vi "Vision Processing.vi"(4 "error in (no error)":errorcluster) -> ()   [LabVIEW 2012]
doc: "This VI runs in parallel to other tasks. It gets images from the camera, processes them for color or shape and use that information to affect robot behavior."
uses:
  Robot Global Data.vi
  Vision Global Data.vi
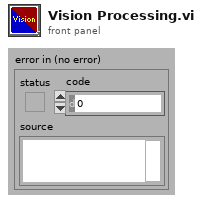
[diagram p1: front panel]
types:
  T1 = typedef "Image Type" = u32
  T2 = typedef "WPI_CameraDevRef.ctl" = cluster{"Camera Address":string, "CameraStatus":errorcluster, "Acquire Image Notifier":refnum<notifier>}
  T3 = typedef "IMAQ Image.ctl" = refnum<image>
  T4 = typedef "TargetData.ctl" = cluster{"X":dbl, "Y":dbl, "Z":dbl}
  T5 = typedef "WPI_CameraImageSize.ctl" = enum16{"640x480", "320x240", "160x120"}
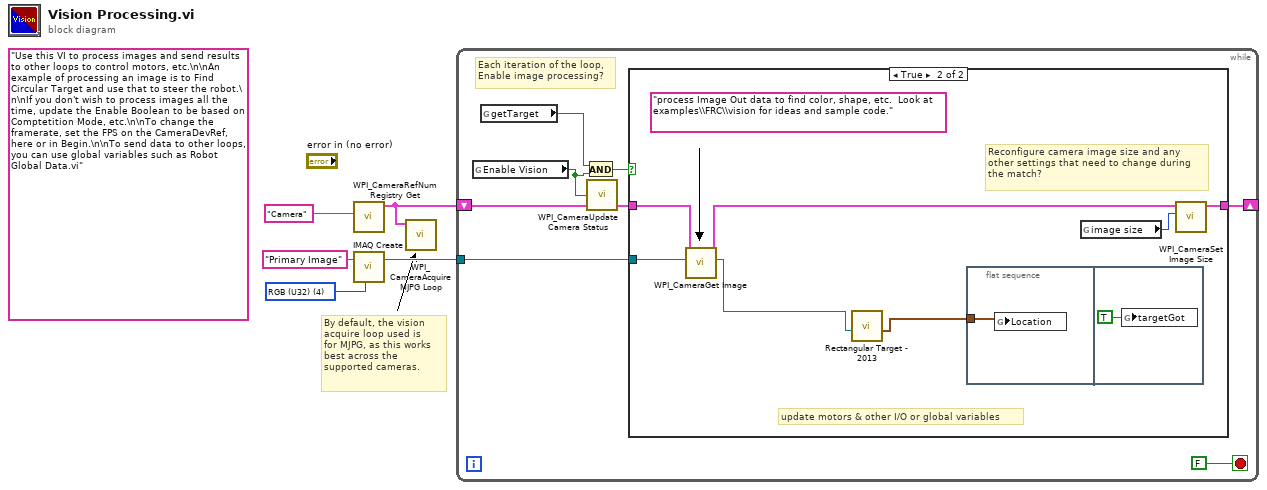
[diagram p0: block diagram]
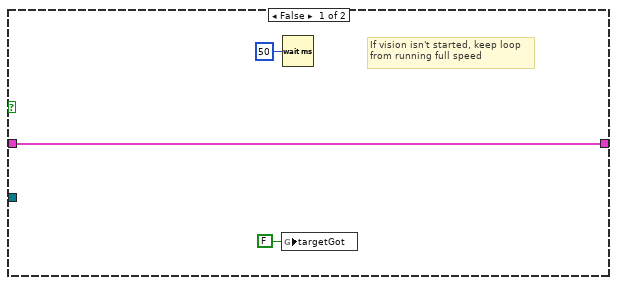
[diagram p2: hidden frame]
diagram:
  (unwired) "Use this VI to process images and send results to other loops to control motors, etc.\n\nAn example of processing an image is to Find Circular Target and use that to steer the robot.\n\nIf you don't wish to process images all the time, update the Enable Boolean to be based on Comptetition Mode, etc.\n\nTo change the framerate, set the FPS on the CameraDevRef, here or in Begin.\n\nTo send data to other loops, you can use global variables such as Robot Global Data.vi"
  w5 = T1 4 items=["Grayscale (U8)", "Grayscale (I16)", "Grayscale (SGL)", "Complex (CSG)", "RGB (U32)", "HSL (U32)", "RGB (U64)"] ("Image Type")
  # "By default, the vision\nacquire loop used is\nfor MJPG, as this works\nbest across the\nsupported cameras."
  n1 = call <vilib>:"WPI_CameraRefNum Registry Get.vi"("refnum name"="Camera") -> ("CameraDevRef"=w1:T2)  [unwired: 1 in, 9 out]
  n2 = call "IMAQ Create"("Image Name"="Primary Image", "Image Type"=w5) -> ("New Image"=w3:T3)  [unwired: 2 in, 2 out]
  n3 = call <vilib>:"WPI_CameraAcquire MJPG Loop.vi"("CameraDevRef"=w1) -> ()  [unwired: 11 in]
  n4 = while {
    shift-right: [w12] -> _
    shift-left: w1 -> [w10]
    tunnel: w3 -> [w11]
    stop <- FALSE stop-if-true
    # "Each iteration of the loop,\nEnable image processing?"
    n5 = global read "Robot Global Data.vi" "Enable Vision"() -> (w6:bool)
    n6 = global read "Vision Global Data.vi" "getTarget"() -> (w7:bool)
    n7 = And(x=w7, y=w6) -> (x .and. y?=w8:bool)
    n8 = call <vilib>:"WPI_CameraUpdate Camera Status.vi"("CameraDevRef In"=w10, "Enable Vision"=w6) -> ("CameraDevRef Out"=w9:T2)  [unwired: 3 in]
    n9 = case shown="True" w8 {
      tunnel: w11 -> [_ w19]
      tunnel: [w16 w23] -> w12
      tunnel: w9 -> [w16 w21]
      frame False {
        # "If vision isn't started, keep loop\nfrom running full speed"
        n10 = global write "Vision Global Data.vi" "targetGot"(FALSE ("targetGot")) -> ()
        n11 = Wait (ms)(milliseconds to wait=u32 50) -> ()  [unwired: 1 out]
      }
      frame True {
        (unwired) "process Image Out data to find color, shape, etc.  Look at examples\\FRC\\vision for ideas and sample code."
        # "update motors & other I/O or global variables"
        # "Reconfigure camera image size and any\nother settings that need to change during\nthe match?"
        n12 = call <vilib>:"WPI_CameraGet Image.vi"("Image"=w19, "CameraDevRef"=w21) -> ("Image Out"=w18:T3, "CameraDevRef Out"=w20:T2)  [unwired: 1 in, 7 out]
        n13 = call "Rectangular Target - 2013.vi"("Original Image 2"=w18) -> ("data"=w17:T4)  [unwired: 10 in]
        n14 = flat-sequence {
          tunnel: w17 -> [w24]
          frame #0 {
            n15 = global write "Vision Global Data.vi" "Location"(w24) -> ()
          }
          frame #1 {
            n16 = global write "Vision Global Data.vi" "targetGot"(TRUE ("targetGot")) -> ()
          }
        }
        n17 = global read "Robot Global Data.vi" "image size"() -> (w22:T5)
        n18 = call <vilib>:"WPI_CameraSet Image Size.vi"("Image Size"=w22, "CameraDevRef"=w20) -> ("CameraDevRef Out"=w23:T2)  [unwired: 1 in, 8 out]
      }
    }
  }
